vi "Sort STEPs.vi"(8 "error in (no error)":errorcluster, 11 "STEPs In":T1[](array[typedef])) -> (0 "error out":errorcluster, 3 "STEPs Out":T1[](array[typedef]))   [LabVIEW 2014, in "SeqLoop.lvlib"]
uses:
  SeqLoop.lvlib
  TypeDefs/STEP.ctl
  TypeDefs/LogicParsedExpression.ctl
  Mimico Display/TypeDefs/Mimic Data.ctl
  Mimico Display/TypeDefs/BG Image.ctl
  Mimico Display/TypeDefs/mObject.ctl
  Mimico Display/Mimico Display.lvlib
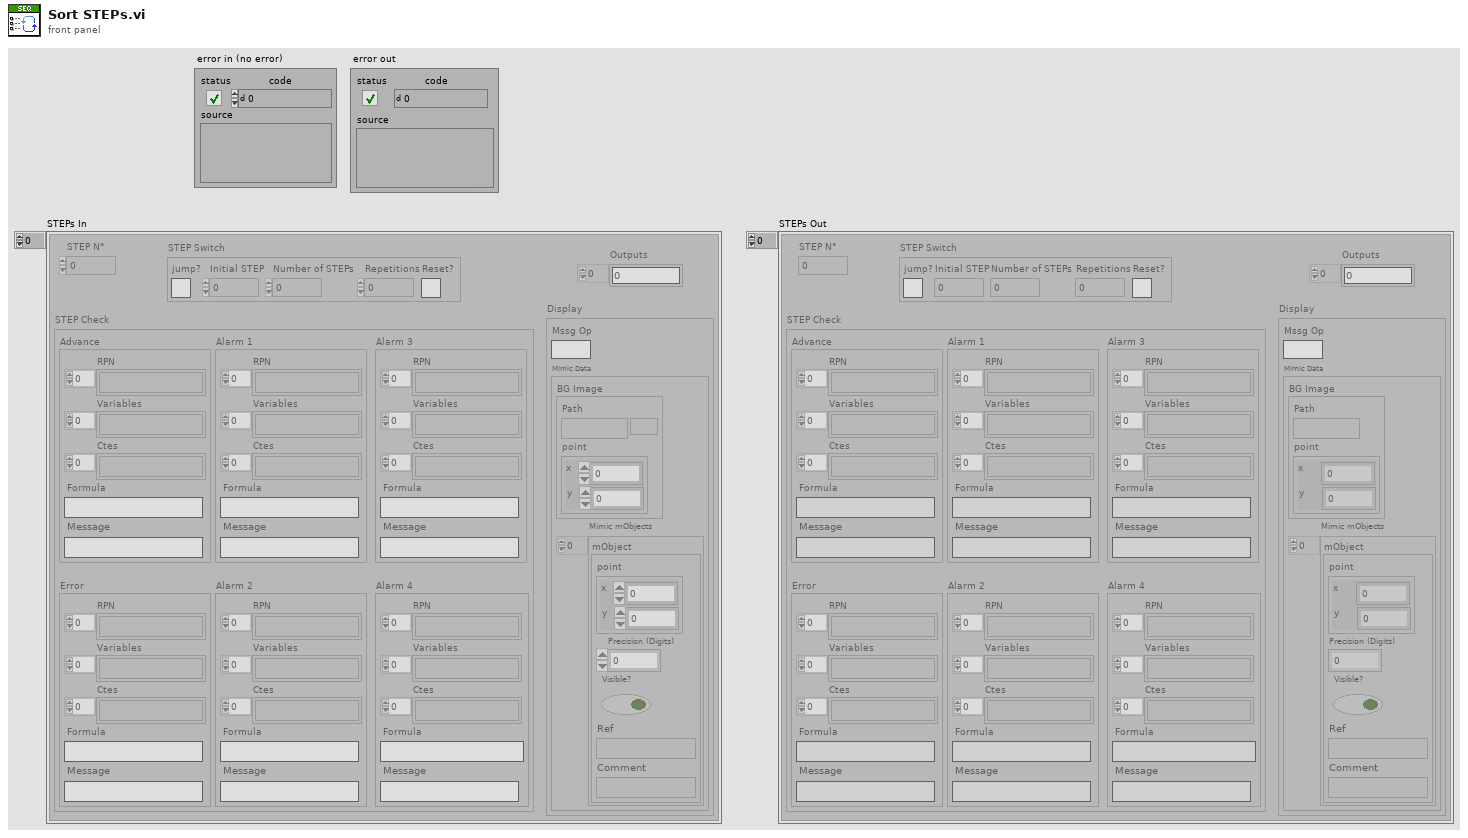
[diagram p1: front panel]
types:
  T1 = typedef "SeqLoop.lvlib/STEP.ctl" = cluster{"STEP N°":u32, "STEP Switch":cluster{"jump?":bool, "Initial STEP":u32, "Number of STEPs":u32, "Repetitions":u32, "Reset?":bool}, "Outputs":i32[], "STEP Check":cluster{"Advance":T2, "Error ":T2, "Alarm 1":T2, "Alarm 2":T2, "Alarm 3":T2, "Alarm 4":T2}, "Display":cluster{"Mssg Op":string, "Mimic Data":T3}}
  T2 = typedef "SeqLoop.lvlib/LogicParsedExpression.ctl" = cluster{"RPN ":string[], "Variables":string[], "Ctes":string[], "Formula":string, "Message":string}
  T3 = typedef "SeqLoop.lvlib/Mimico Display.lvlib/Mimic Data.ctl" = cluster{"BG Image":T4, "Mimic mObjects":T5[]}
  T4 = typedef "SeqLoop.lvlib/Mimico Display.lvlib/BG Image.ctl" = cluster{"Path":path, "point":cluster{"x":i16, "y":i16}}
  T5 = typedef "SeqLoop.lvlib/Mimico Display.lvlib/mObject.ctl" = cluster{"point":cluster{"x":i16, "y":i16}, "Precision (Digits)":i32, "Visible?":bool, "Ref":string, "Comment":string}
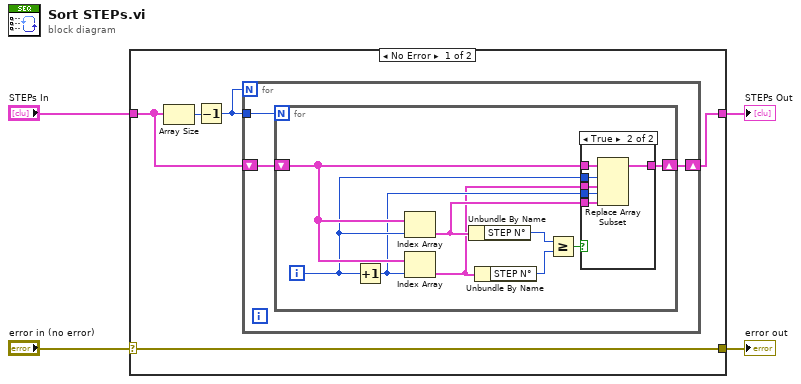
[diagram p0: block diagram]
diagram:
  n1 = case shown="No Error" "error in (no error)" {
    selector: "error in (no error)" -> [w5 w29]
    tunnel: "STEPs In" -> [w7 w30]
    tunnel: [w6 w30] -> w1
    tunnel: [w5 w29] -> w4
    frame No Error {
      n2 = Array Size(array=w7) -> (size(s)=w9:i32)
      n3 = Decrement(x=w9) -> (x-1=w8:i32)
      n4 = for {
        N: w8 -> [_]
        shift-right: [w11] -> w6
        shift-left: w7 -> [w12]
        tunnel: w8 -> [w10]
        n5 = for {
          N: w10 -> [_]
          shift-right: [w20] -> w11
          shift-left: w12 -> [w19]
          i -> [w18]
          n6 = Increment(x=w18) -> (x+1=w17:i32)
          n7 = Index Array(array=w19, index=w18) -> (element=w16:T1)
          n8 = Index Array(array=w19, index=w17) -> (element=w14:T1)
          n9 = Unbundle By Name(w16) -> ("STEP N°"=w15:u32)
          n10 = Unbundle By Name(w14) -> ("STEP N°"=w13:u32)
          n11 = Greater Or Equal?(x=w15, y=w13) -> (x >= y?=w21:bool)
          n12 = case shown="True" w21 {
            tunnel: [w22 w28] -> w20
            tunnel: w19 -> [w22 w27]
            tunnel: w16 -> [_ w26]
            tunnel: w14 -> [_ w25]
            tunnel: w18 -> [_ w24]
            tunnel: w17 -> [_ w23]
            frame False {
            }
            frame True {
              n13 = Replace Array Subset(array=w27, new element #1=w25, index #1=w24, new element #2=w26, index #2=w23) -> (w28:T1[])
            }
          }
        }
      }
    }
    frame Error {
    }
  }
  "error out" <- w4
  "STEPs Out" <- w1
